vi "Set LVCompare Options.vi"(8 "error in":errorcluster, 9 "TimeOut on Error (250ms)":i32=250, 10 "Retries (10)":i32=10, 11 "compare options (All True)":T1={"VI Attributes"=TRUE, "Front Panel"=TRUE, "FP position/size"=TRUE, "Block Diagram"=TRUE, "BD cosmetic"=TRUE, "BD position/size"=TRUE}) -> (0 "error out":errorcluster)   [LabVIEW 2020, in "Approval Tests.lvlib"]
uses:
  Approval Tests.lvlib
  LVCompare Options.ctl
  Global.vi
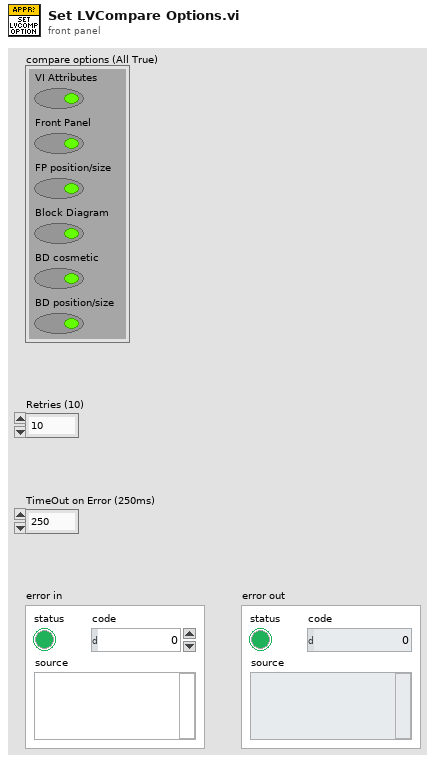
[diagram p1: front panel]
types:
  T1 = typedef "Approval Tests.lvlib/LVCompare Options.ctl" = cluster{"VI Attributes":bool, "Front Panel":bool, "FP position/size":bool, "Block Diagram":bool, "BD cosmetic":bool, "BD position/size":bool}
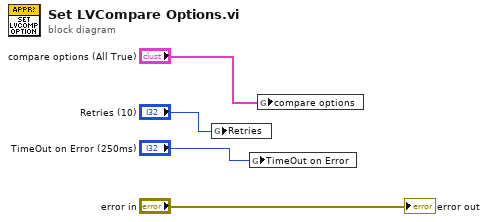
[diagram p0: block diagram]
diagram:
  n1 = global write "Global.vi" "Retries"("Retries (10)") -> ()
  n2 = global write "Global.vi" "TimeOut on Error"("TimeOut on Error (250ms)") -> ()
  n3 = global write "Global.vi" "compare options"("compare options (All True)") -> ()
  "error out" <- "error in"
